vi "getSenMfileName.vi"(8 "error in (no error)":errorcluster, 10 "Regular Expression":string="\\AsenM\\S+", 11 "OptStateEsti in":refnum<class "OptStateEsti.lvclass">) -> (0 "error out":errorcluster, 2 "Sen M File Name":string="senM_35_19_50.txt", 3 "OptStateEsti out":refnum<class "OptStateEsti.lvclass">)   [LabVIEW 2016, in "OfcFunc.lvlib" / "OptStateEsti.lvclass"]
doc: "Get the sensitivity matrix M file name."
uses:
  OptStateEsti.lvclass
  OptStateEsti.lvclass/OptStateEsti.ctl
  <vilib>/regexp/Match Regular Expression.xnode
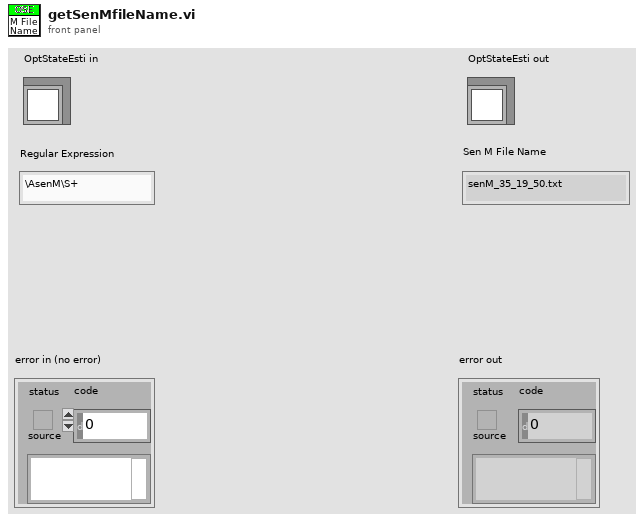
[diagram p1: front panel]
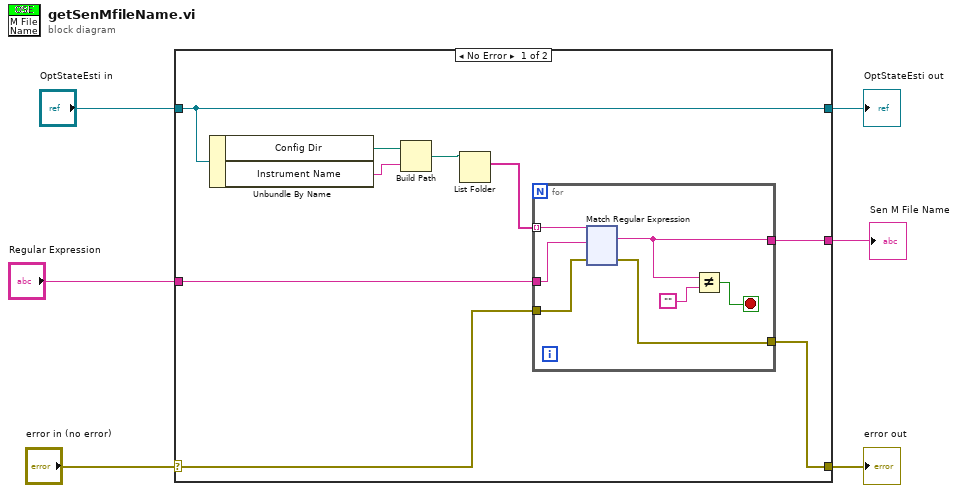
[diagram p0: block diagram]
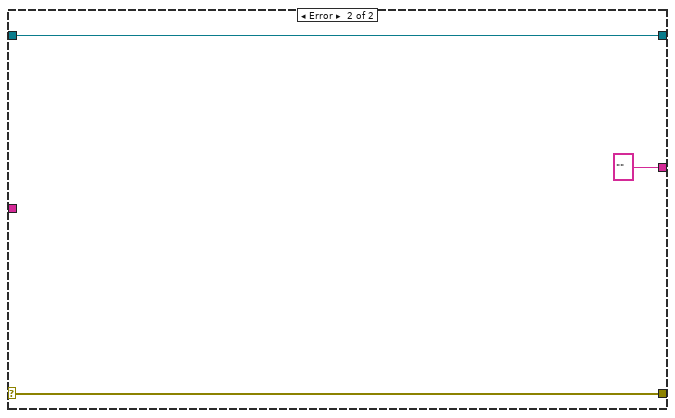
[diagram p2: hidden frame]
diagram:
  n1 = case shown="No Error" "error in (no error)" {
    selector: "error in (no error)" -> [w8 w137]
    tunnel: [w7 w137] -> w5
    tunnel: [w15 w139] -> w3
    tunnel: "OptStateEsti in" -> [w15 w139]
    tunnel: [w9 ""] -> w2
    tunnel: "Regular Expression" -> [w10 _]
    frame No Error {
      n2 = Unbundle By Name(w15) -> ("Config Dir"=w14:path, "Instrument Name"=w13:string)
      n3 = Build Path(base path=w14, name or relative path=w13) -> (appended path=w12:path)
      n4 = List Folder(path=w12) -> (filenames=w11:string[])  [unwired: 3 in, 3 out]
      n5 = for {
        tunnel: w11 -> [w22] mode=indexing
        tunnel: w10 -> [w21]
        tunnel: [w18] -> w9
        tunnel: w8 -> [w17]
        tunnel: [w16] -> w7
        stop <- w19 stop-if-true
        n6 = xnode "Match Regular Expression"("input string"=w22, "regular expression"=w21, "error in"=w17) -> ("whole match"=w18:string, "error out"=w16:errorcluster)  [unwired: 3 in, 3 out]
        n7 = Not Equal?(x=w18, y="") -> (x != y?=w19:bool)
      }
    }
    frame Error {
    }
  }
  "error out" <- w5
  "OptStateEsti out" <- w3
  "Sen M File Name" <- w2
